vi "Positions.vi"() -> ()   [LabVIEW 2018]
panel:
  in  "Custom Elevator Speed":dbl=1000.0
  in  "Intake Out":dbl=1.0
  in  "Intake In":dbl=-1.0
  in  "Shooter Out":dbl=-1.0
  in  "Shooter In":dbl=1.0
  in  "Pivot Second Level":dbl=800.0
  in  "Elevator Cargoship":dbl=10500.0
  in  "Elevator First Level":dbl=5500.0
  in  "Pivot Under Flat":dbl=1300.0
  in  "Climber 90*":dbl=2000.0
  in  "Climber Climb":dbl=5500.0
  in  "Elevator Tucked":dbl=500.0
  in  "Pivot Up":dbl
  in  "Elevator Intake":dbl=500.0
  in  "Climber Clear":dbl=1500.0
  in  "Elevator Clearance":dbl=4750.0
  in  "Pivot Intake":dbl=1650.0
  in  "Elevator Second level":dbl=15000.0
  in  "First Ball":dbl=7500.0
  in  "Climber Intake":dbl=2700.0
  in  "Climber Up":dbl=100.0
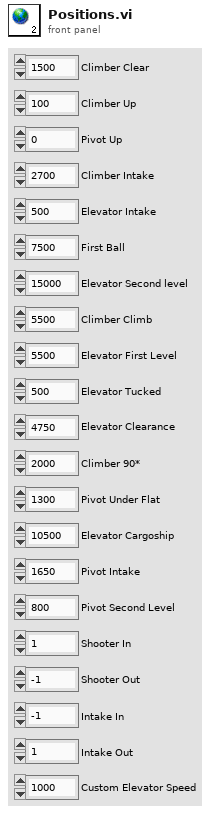
[diagram p1: front panel]
diagram:
